vi "writeToXML.vi"(8 "error in (no error)":errorcluster, 10 "ClassLabel":string, 11 "RotCurrentWrap in":refnum<class "RotCurrentWrap.lvclass">) -> (0 "error out":errorcluster, 2 "XML out":string, 3 "RotCurrentWrap out":refnum<class "RotCurrentWrap.lvclass">)   [LabVIEW 2014, in "TCSDataDefinitions.lvlib" / "TCSCommand.lvlib" / "CableWrapCommands.lvlib" / "RotCurrentWrap.lvclass"]
uses:
  RotCurrentWrap.lvclass
  CableWrapCommands/CableWrapCommands.lvclass
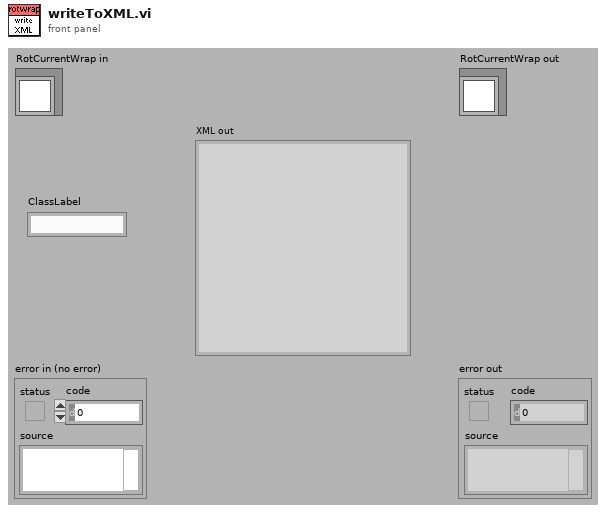
[diagram p1: front panel]
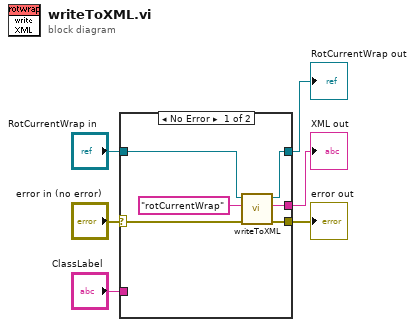
[diagram p0: block diagram]
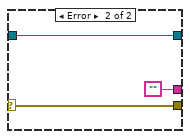
[diagram p2: hidden frame]
diagram:
  n1 = case shown="No Error" "error in (no error)" {
    selector: "error in (no error)" -> [w8 w14]
    tunnel: [w12 w14] -> w6
    tunnel: [w11 ""] -> w5
    tunnel: [w10 w15] -> w4
    tunnel: "RotCurrentWrap in" -> [w9 w15]
    tunnel: "ClassLabel" -> [_ _]
    frame No Error {
      n2 = call-parent "writeToXML.vi"("error in (no error)"=w8, "Class Label"="rotCurrentWrap", "CableWrapCommands in"=w9) -> ("error out"=w12:errorcluster, "XML out"=w11:string, "CableWrapCommands out"=w10:refnum<class "RotCurrentWrap.lvclass">)  [unwired: 6 out]
    }
    frame Error {
    }
  }
  "error out" <- w6
  "RotCurrentWrap out" <- w4
  "XML out" <- w5
